vi "220929_MathNode.vi"() -> ()   [LabVIEW 2022 SP3]
uses:
  <vilib>/numeric/Random Number (Range) U64.vi
  <vilib>/numeric/sub_Random U32.vi
panel:
  out "Pt100":cluster{u64[], dbl[]}(graph)
  out "T in Grad":dbl[](array[numeric])
  in  "R0":dbl
  in  "A-const.":dbl=-5.7e-07
  in  "B-const.":dbl=0.0039
  in  "Wertvalue":i32
  out "R in Ohm":u64[](array[numeric])
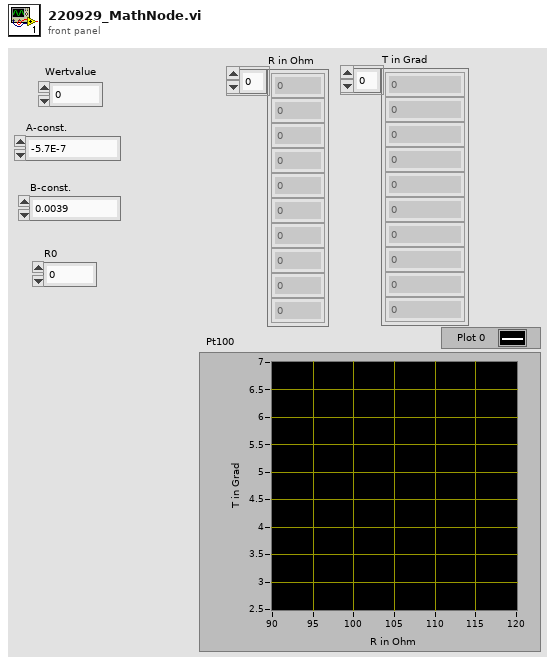
[diagram p1: front panel]
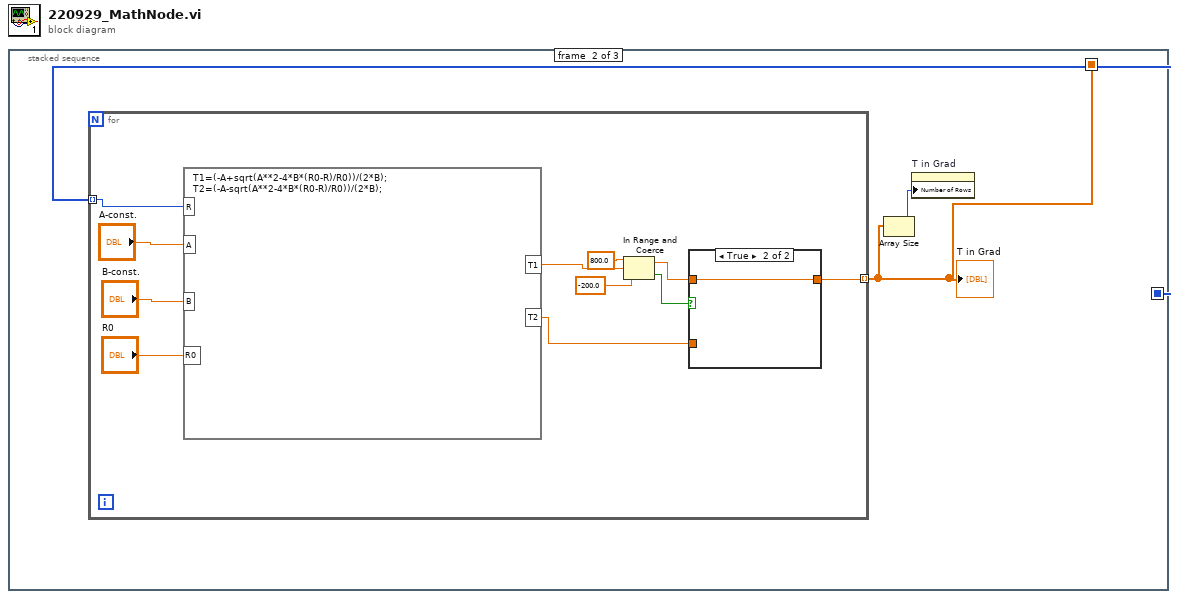
[diagram p0: block diagram]
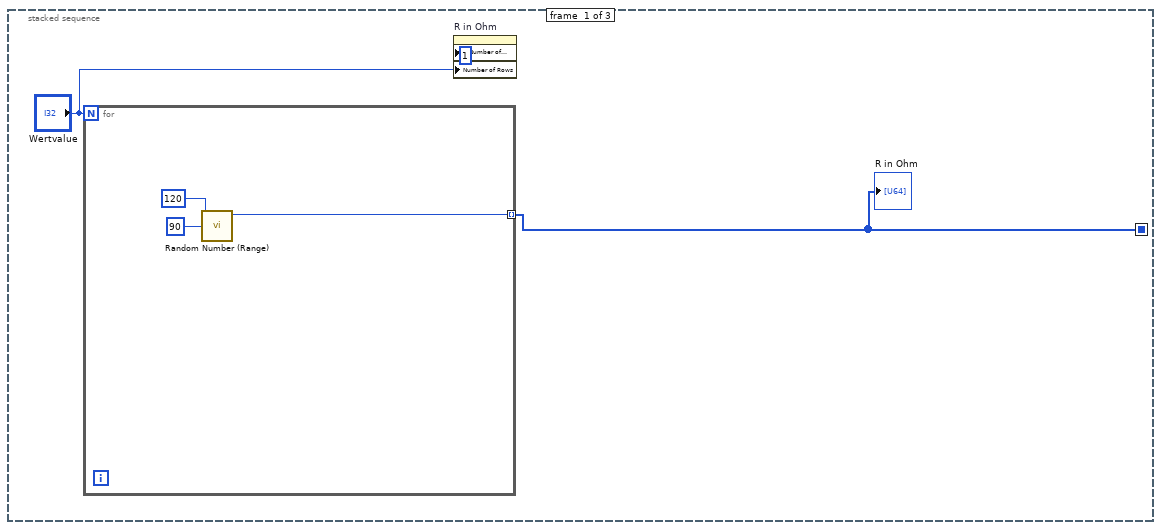
[diagram p2: hidden frame]
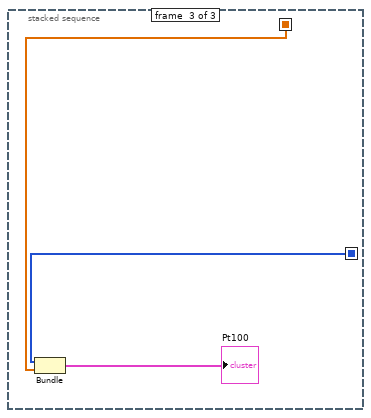
[diagram p4: hidden frame]
diagram:
  n1 = stacked-sequence {
    seq-local: [w3 _ _] -> [_ w9 w25]
    seq-local: [_ w7 _] -> [_ _ w24]
    frame #0 {
      n2 = for {
        N: "Wertvalue" -> [_]
        tunnel: [w4] -> w3 mode=indexing
        n3 = call-poly <vilib>:"Random Number (Range).vi"("lower bound (0)"=u64 90, "upper bound (100)"=u64 120) -> ("number"=w4:u64)  [unwired: 9 in]
      }
      "R in Ohm" <- w3
      n4 = property on="R in Ohm" class="Arr (strict)"("Number of Columns"=u32 1, "Number of Rows"="Wertvalue") -> ()  [unwired: 2 in, 2 out]
    }
    frame #1 {
      n5 = for {
        tunnel: w9 -> [w20] mode=indexing
        tunnel: [w12] -> w7 mode=indexing
        n6 = formula code="T1=(-A+sqrt(A**2-4*B*(R0-R)/R0))/(2*B);\nT2=(-A-sqrt(A**2-4*B*(R0-R)/R0))/(2*B);"("R"=w20, "A"="A-const.", "B"="B-const.", "R0"="R0") -> ("T1"=w11:dbl, "T2"=w10:dbl)
        n7 = In Range and Coerce(upper limit=800.0, x=w11, lower limit=-200.0) -> (coerced(x)=w13:dbl, In Range?=w14:bool)
        n8 = case shown="True" w14 {
          tunnel: w13 -> [_ w22]
          tunnel: [w21 w22] -> w12
          tunnel: w10 -> [w21 _]
          frame False {
          }
          frame True {
          }
        }
      }
      "T in Grad" <- w7
      n9 = Array Size(array=w7) -> (size(s)=w8:i32)
      n10 = property on="T in Grad" class="Arr (strict)"("Number of Rows"=w8) -> ()  [unwired: 2 in, 2 out]
    }
    frame #2 {
      n11 = Bundle(w25, w24) -> (→"Pt100":cluster{u64[], dbl[]})  [unwired: 1 in]
    }
  }
